vi "Drive Controller.vi"(8 "error in":errorcluster) -> ()   [LabVIEW 2018]
doc: "This VI executes continuously carrying out the current operation and responding to updates or new operation requests. It will often contain the timing or control code that is difficult to place directly in TeleOp. This VI generally opens all sensors and motors and isolates the rest of the robot code from knowing implementation details of how the operations are carried out."
uses:
  <vilib>/Rock Robotics/WPI/Framework/Completion Status.ctl
  Drive Setpoints.ctl
  Drive Operations.ctl
  Dawgma Programming Library/Controls/PurePursuit/RobotNeededPathData.ctl
  <vilib>/Rock Robotics/WPI/SafetyOutput/WPI_SafetyOutputConfigMenu.ctl
  <vilib>/Rock Robotics/SystemInterfaces/DIO/FPGA_DIOPWMChannel.ctl
  <vilib>/Rock Robotics/SystemInterfaces/DIO/FPGA_DIOChannel.ctl
  Logging/DataNames.ctl
  <vilib>/Rock Robotics/WPI/DriverStation/WPI_DriverStationRobotMode2.ctl
  <extravilib>/ChannelInstances/Lossy Stream-c(dbl,dbl,dbl,c(dbl,dbl))/Write With Abort.vi
  <extravilib>/ChannelInstances/Lossy Stream-c(dbl,dbl,dbl,c(dbl,dbl))/Read With Abort.vi
  <extravilib>/ChannelInstances/Lossy Stream-c(dbl,dbl,dbl,c(dbl,dbl))/Endpoint.vi
  <extravilib>/ChannelInstances/Lossy Stream-c(dbl,dbl,dbl,c(dbl,dbl))/EndpointRead.vi
  <vilib>/Rock Robotics/WPI/RobotDrive/WPI_RobotDriveOpen4MotorWithSPARK.vi
  <vilib>/Rock Robotics/WPI/Counter/WPI_CounterDigitalInputToDigitalSource.vi
  <vilib>/Rock Robotics/WPI/RobotDrive/WPI_RobotDriveOpen2MotorWithSPARK.vi
  <extravilib>/ChannelInstances/Lossy Stream-c(dbl,dbl,dbl,c(dbl,dbl))/Instantiate.vi
  Framework/Robot Global Data.vi
  <extravilib>/ChannelInstances/Lossy Stream-c(dbl,dbl,dbl,c(dbl,dbl))/)Channel.vi
  <resource>/ChannelSupport/_ChannelSupport/WaitIfNeeded.vi
  <vilib>/addons/control/pid/pid.llb/PID (DBL).vi
  Configuration/Constants.vi
  Drive Published Globals.vi
  <vilib>/Rock Robotics/Network Tables/NT Read Number.vi
  <vilib>/Rock Robotics/Network Tables/NT Write Number.vi
  <vilib>/addons/control/pid/NI_PID_pid.lvlib
  <extravilib>/ChannelInstances/Lossy Stream-c(dbl,dbl,dbl,c(dbl,dbl)).lvlib
panel:
  in  "Integral Range":dbl=15.0
  out "PID Tuining":cluster{dbl, dbl}(graph)={170.0, 167.02}
  in  "Points":cluster{"X":dbl, "Y":dbl}[](array[cluster])=[{"X"=0.0, "Y"=0.0}, {"X"=0.01, "Y"=0.0}, {"X"=0.011, "Y"=0.17}, {"X"=1.0, "Y"=1.0}]
  in  "PID gains":T1={"proportional gain (Kc)"=0.01, "integral time (Ti, min)"=0.007, "derivative time (Td, min)"=0.0015} {"derivative time (Td, min)" format="%#_9g"}
  in  "Gains":T2={"FFV"=0.0059, "FFA"=0.0019, "Vel PID"={"P"=0.01, "I"=0.0, "D"=0.0}}
  in  "Interactive Values":T3={"Operation"=enum."Turn to Angle", "Left Speed"=-0.27, "Right Speed"=0.27, "Duration"=2.0, "Speed"=0.0, "Start Angle"=0.0, "Target Angle"=180.0, "Distance (inch)"=0.0, "Start Point (inch)"=0.0, "RobotNeededPathData"={"Path"=[], "MaxVel"=0.0, "MaxAccel"=-1.0, "Backwards?"=FALSE, "PointSpacing"=0.0, "LookaheadDist"=0.0, "Speed/Curve"=1.8, "SlowDistanceAtEnd"=12.0, "SlowSpeed"=15.0, "MaxDeAccel"=0.0}, "Start Point 2"=0.0} {"RobotNeededPathData"."SlowSpeed" format="%#_13g"; "RobotNeededPathData"."SlowDistanceAtEnd" format="%#_13g"; "RobotNeededPathData"."Speed/Curve" format="%#_13g"}
  in  "Buttons":cluster{"Execute Cmd":bool, "Abort Cmd":bool}
  out "Command Timing":cluster{"Start Time (ms)":u32, "Iterations":i32}={"Start Time (ms)"=372507, "Iterations"=0}
  out "Status":T6
  out "Setpoints":T7(graph)
  out "Current\nCmd":string="Started at  14:51:47.884\nDefault: Reserve,  L 0.0, R 0.0, D 0.000000"
  # "Tip: The graph shows the motor setpoints. It may also be helpful to observe inputs and sensor values.\nYou may also want to display tuning or debugging controls."
  # "Interactive Command: You may fill in the settings for a command\nand schedule it with the Execute button. You can observe and abort\nany command while fine tuning the code for the controller."
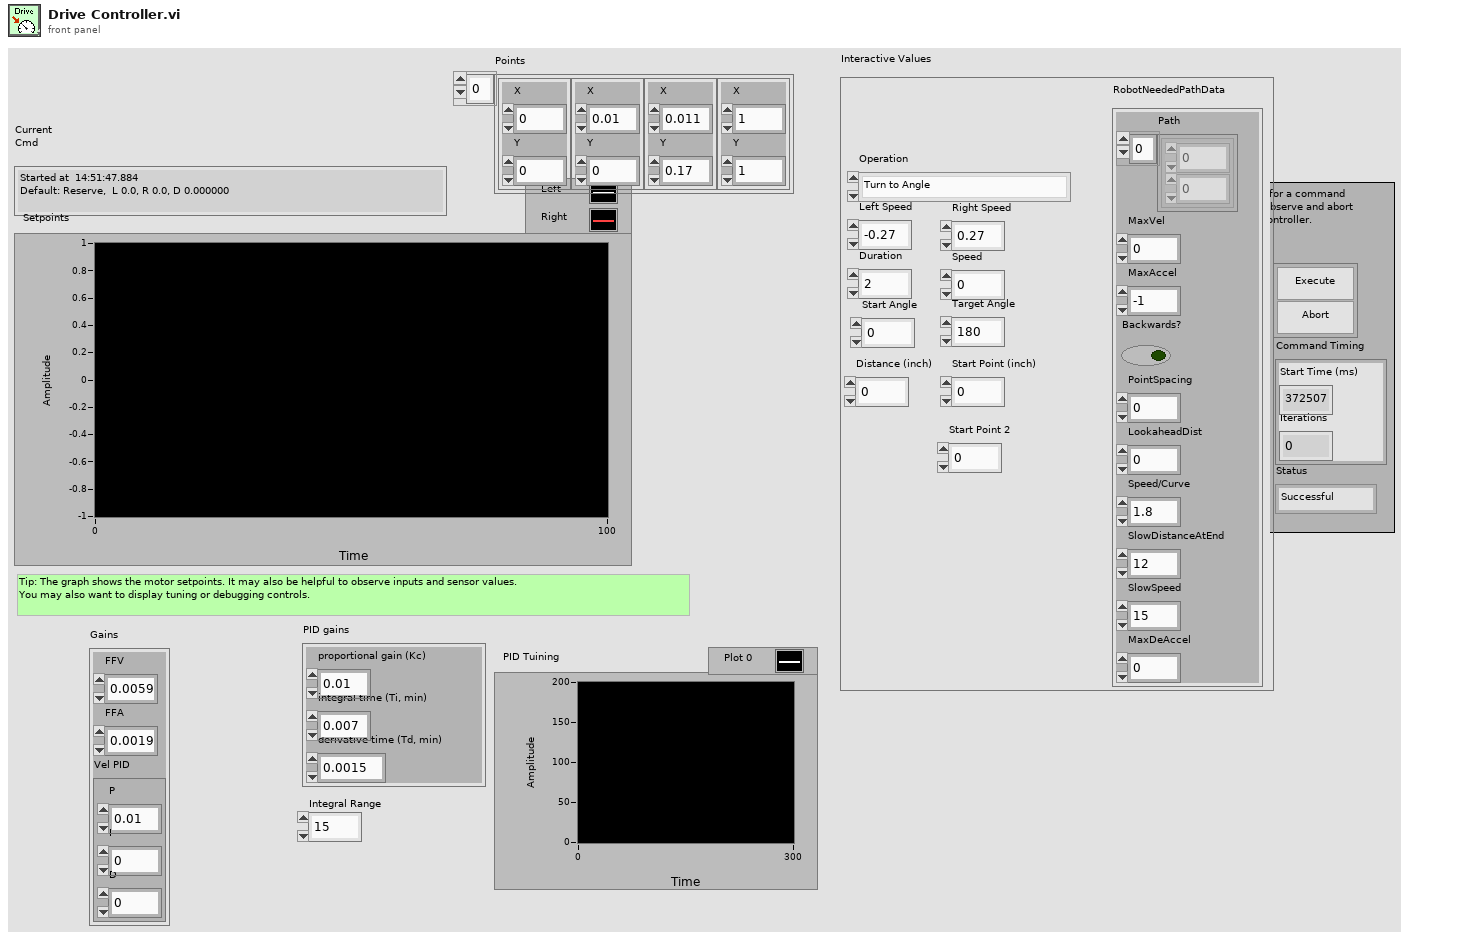
[diagram p1: front panel]
types:
  T1 = cluster{"proportional gain (Kc)":dbl, "integral time (Ti, min)":dbl, "derivative time (Td, min)":dbl}
  T2 = cluster{"FFV":dbl, "FFA":dbl, "Vel PID":cluster{"P":dbl, "I":dbl, "D":dbl}}
  T3 = typedef "Drive Setpoints.ctl" = cluster{"Operation":T4, "Left Speed":dbl, "Right Speed":dbl, "Duration":dbl, "Speed":dbl, "Start Angle":dbl, "Target Angle":dbl, "Distance (inch)":dbl, "Start Point (inch)":dbl, "RobotNeededPathData":T5, "Start Point 2":dbl}
  T4 = typedef "Drive Operations.ctl" = enum16{"Reserve", "Read Current", "Immediate", "Drive for Time", "Drive for Distance", "Turn to Angle", "Drive Path"}
  T5 = typedef "RobotNeededPathData.ctl" = cluster{"Path":cluster{dbl, dbl}[], "MaxVel":dbl, "MaxAccel":dbl, "Backwards?":bool, "PointSpacing":dbl, "LookaheadDist":dbl, "Speed/Curve":dbl, "SlowDistanceAtEnd":dbl, "SlowSpeed":dbl, "MaxDeAccel":dbl}
  T6 = typedef "Completion Status.ctl" = enum16{"Successful", "Aborted", "Incomplete"}
  T7 = cluster{"Left Setpoint":dbl, "Right Setpoint":dbl}
  T8 = typedef "DataNames.ctl" = enum16{"RobotMode", "FMSConnected", "DriveLeft", "DriveRight", "EncoderLeft", "EncoderRight", "Angle", "LocationX", "LocationY", "CPU", "DriveOperation", "Battery"}
  T9 = typedef "FPGA_DIOChannel.ctl" = enum8{"DIO 0", "DIO 1", "DIO 2", "DIO 3", "DIO 4", "DIO 5", "DIO 6", "DIO 7", "DIO 8", "DIO 9", "DIO MXP 0", "DIO MXP 1", "DIO MXP 2", "DIO MXP 3", "DIO MXP 4", "DIO MXP 5", "DIO MXP 6", "DIO MXP 7", "DIO MXP 8", "DIO MXP 9", "DIO MXP 10", "DIO MXP 11", "DIO MXP 12", "DIO MXP 13", "DIO MXP 14", "DIO MXP 15", "SPI Port CS1", "SPI Port CS2", "SPI Port CS3", "SPI Port MISO", "SPI Port MOSI", "Invalid"}
  T10 = typedef "FPGA_DIOPWMChannel.ctl" = enum8{"PWM 0", "PWM 1", "PWM 2", "PWM 3", "PWM 4", "PWM 5", "PWM 6", "PWM 7", "PWM 8", "PWM 9", "PWM MXP 0", "PWM MXP 1", "PWM MXP 2", "PWM MXP 3", "PWM MXP 4", "PWM MXP 5", "PWM MXP 6", "PWM MXP 7", "PWM MXP 8", "PWM MXP 9", "Invalid"}
  T11 = typedef "WPI_SafetyOutputConfigMenu.ctl" = enum16{"Enable", "Disable"}
  T12 = typedef "WPI_DigitalInputDevRef.ctl" = cluster{"DevStatus":errorcluster, "DIO Channel":T9}
  T13 = typedef "FPGA_CounterEncoderSourceConvertionLVSourceType.ctl" = cluster{"DevStatus":errorcluster, "AnalogTriggerMode?":bool, "DigitalMode":cluster{"DIO Channel":T14}, "AnalogTriggerMode":cluster{"AnalogTriggerIndex":T15, "OutputType":T16}}
  T14 = typedef "FPGA_DIODigitalSourceChannel.ctl" = enum8{"DIO 0", "DIO 1", "DIO 2", "DIO 3", "DIO 4", "DIO 5", "DIO 6", "DIO 7", "DIO 8", "DIO 9", "DIO MXP 0", "DIO MXP 1", "DIO MXP 2", "DIO MXP 3", "DIO MXP 4", "DIO MXP 5", "DIO MXP 6", "DIO MXP 7", "DIO MXP 8", "DIO MXP 9", "DIO MXP 10", "DIO MXP 11", "DIO MXP 12", "DIO MXP 13", "DIO MXP 14", "DIO MXP 15", "SPI Port CS1", "SPI Port CS2", "SPI Port CS3", "SPI Port MISO", "SPI Port MOSI", "Disabled"}
  T15 = typedef "FPGA_AnalogTriggerIndex.ctl" = enum8{"Trig 0", "Trig 1", "Trig 2", "Trig 3", "Trig 4", "Trig 5", "Trig 6", "Trig 7", "Invalid"}
  T16 = typedef "FPGA_AnalogTriggerOutType.ctl" = enum16{"InWindow", "TriggerState", "Rising", "Falling"}
  T17 = typedef "WPI_EncoderDevRef.ctl" = cluster{"DevStatus":errorcluster, "EncoderIndex":T18, "CounterIndex":T19, "DistancePerCount":dbl, "Decoding Type":T20}
  T18 = typedef "FPGA_EncoderIdx.ctl" = enum8{"Enc 0", "Enc 1", "Enc 2", "Enc 3", "Enc 4", "Enc 5", "Enc 6", "Enc 7", "Invalid"}
  T19 = typedef "FPGA_CounterCtrSystemIndex.ctl" = enum8{"Ctr 0", "Ctr 1", "Ctr 2", "Ctr 3", "Ctr 4", "Ctr 5", "Ctr 6", "Ctr 7", "Invalid"}
  T20 = typedef "WPI_EncoderType.ctl" = enum16{"1x", "2x", "4x"}
  T21 = typedef "WPI_RobotDriveDevRef.ctl" = cluster{"DevStatus":errorcluster, "Motors[]":T22[], "Square Inputs":bool, "Max Output":dbl}
  T22 = typedef "WPI_MotorControlDeviceRef.ctl" = cluster{"DeviceStatus":errorcluster, "Type":T23, "PWM":cluster{"PWM Channel":T10, "DeadBand":T24}, "CAN":cluster{"Device Number":u8, "SetOutput VI Ref":variant, "GetOutput VI Ref":variant, "Enable VI Ref":variant, "Disable VI Ref":variant, "Data":variant}, "Invert":bool, "DIO PWM":cluster{"PWM \"Enable\" Channel":T10, "DIOChannel":T9, "PWM Rate":dbl}}
  T23 = typedef "WPI_MotorControlType.ctl" = enum16{"PWM", "CAN", "DIO PWM"}
  T24 = typedef "WPI_PWMDeadband.ctl" = cluster{"Name":string, "maxPositivePwm":i32, "minPositivePwm":i32, "centerPwm":i32, "maxNegativePwm":i32, "minNegativePwm":i32, "angularRange":u16}
  T25 = typedef "Command Status Info.ctl" = cluster{"Name":string, "Status":T6, "notifier out":T26}
  T26 = typedef "Completion Notifier.ctl" = refnum<notifier>
  T27 = cluster{"SubSystem Data":T3, cluster{"Start Time (ms)":u32, "Iterations":i32}, cluster{"Command Info":T25, "Description":string, "Default Command":T3, "queue out":refnum<queue>, "Subsystem Name":string}}
  T28 = cluster{"LeftVel":dbl, "RightVel":dbl, "Yaw":dbl, "Pos":cluster{"X":dbl, "Y":dbl}}
  T29 = typedef "WPI_DriverStationRobotMode2.ctl" = enum16{"Autonomous Disabled", "Autonomous Enabled", "Teleop Disabled", "Teleop Enabled", "Disconnected", "Finish", "Test Disabled", "Test Enabled", "Emergency Stopped"}
  T30 = cluster{"Yaw":dbl, "Roll":dbl, "Pitch":dbl, "Heading":dbl, "Fused Heading":dbl}
  T31 = typedef "Lossy Stream-c(dbl,dbl,dbl,c(dbl,dbl)).lvlib/)Channel.ctl" = refnum<queue>
  T32 = cluster{"LeftDistance":dbl, "RightDistance":dbl, "LeftVelocity":dbl, "RightVelocity":dbl, "Angle":dbl, "Location":cluster{dbl, dbl}}
  T33 = cluster{"dx/dt":dbl, "dx/dt":dbl, "Yaw":dbl, cluster{dbl, dbl}}
  T34 = cluster{"SubSystem Data":T3, cluster{"Start Time (ms)":u32, "Iterations":i32}, "Default Command Arguments":cluster{"Command Info":T25, "Description":string, "Default Command":T3, "queue out":refnum<queue>, "Subsystem Name":string}}
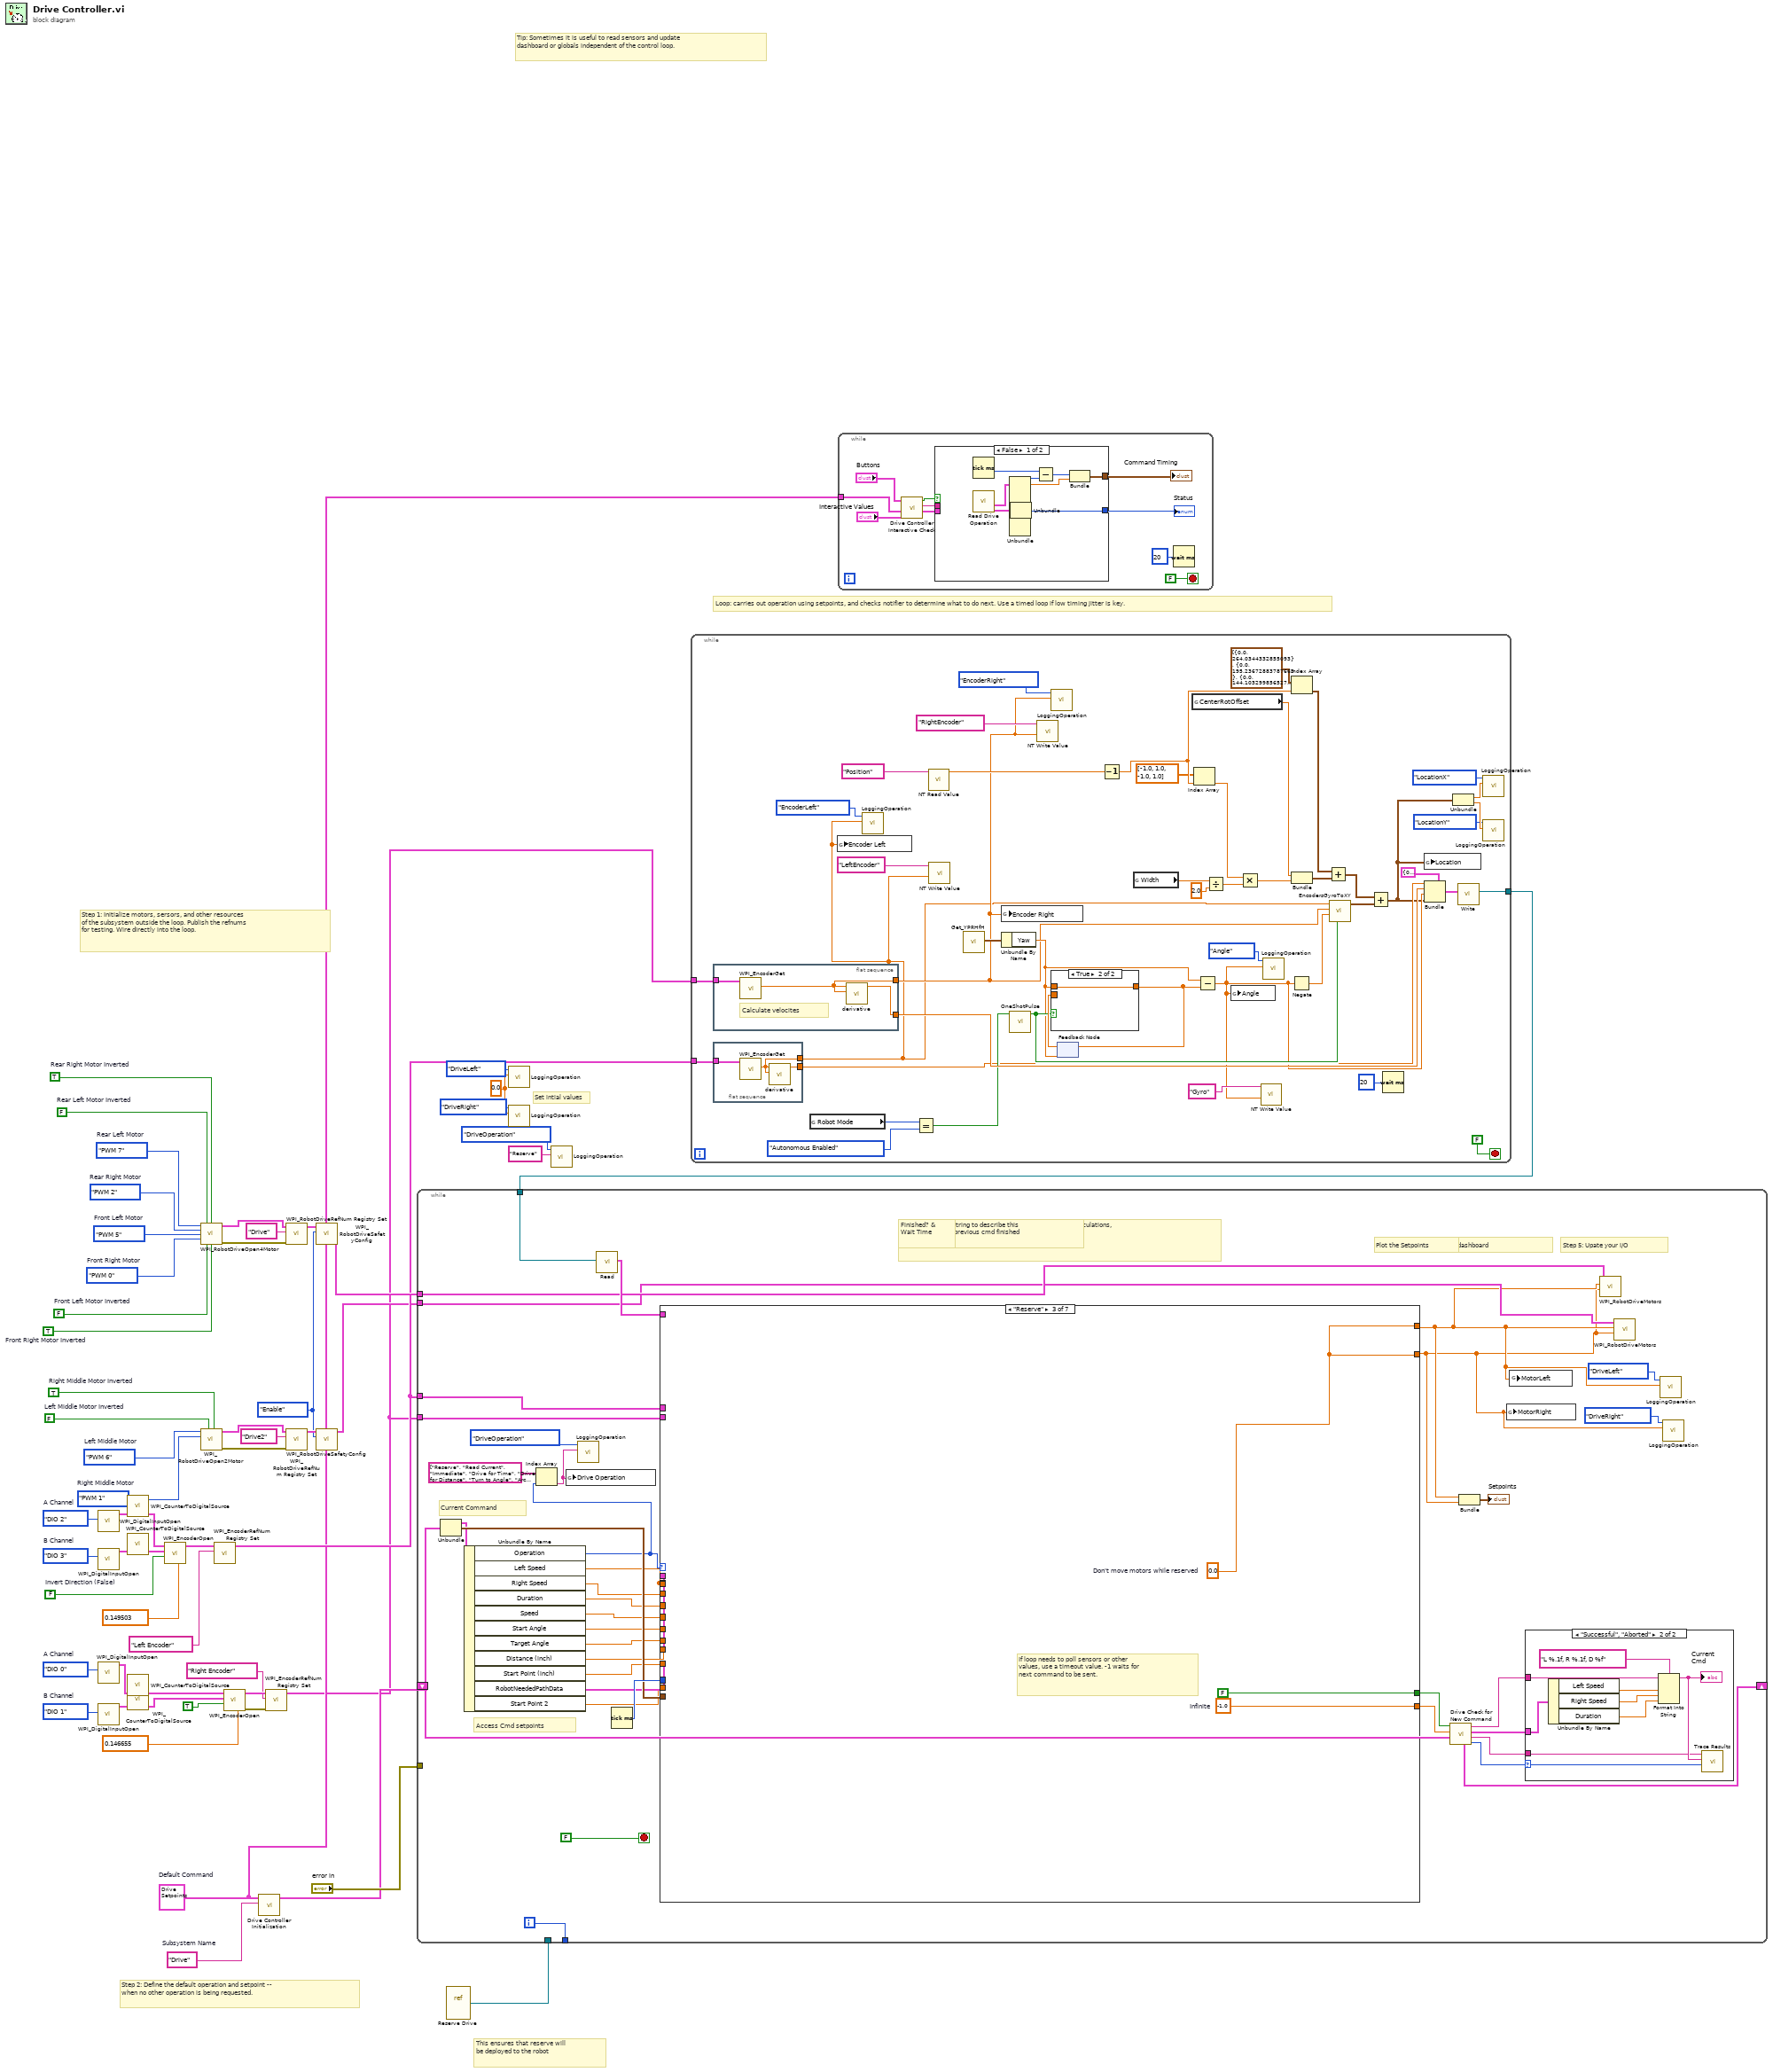
[diagram p0: block diagram]
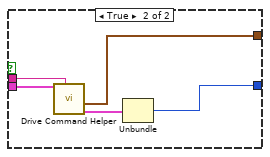
[diagram p3: hidden frame]
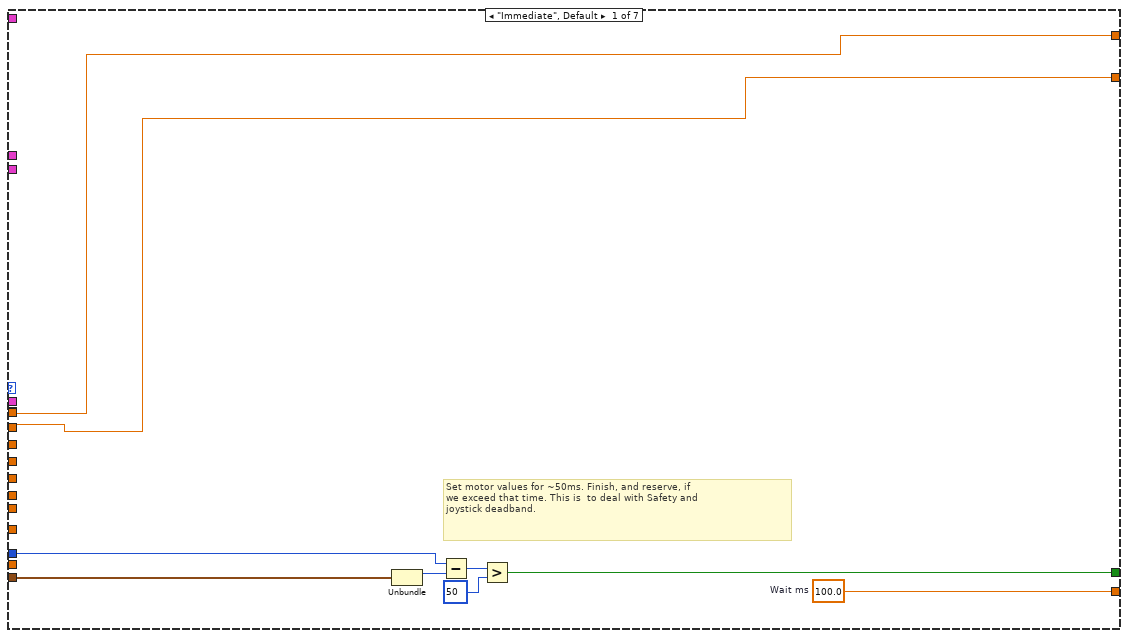
[diagram p4: hidden frame]
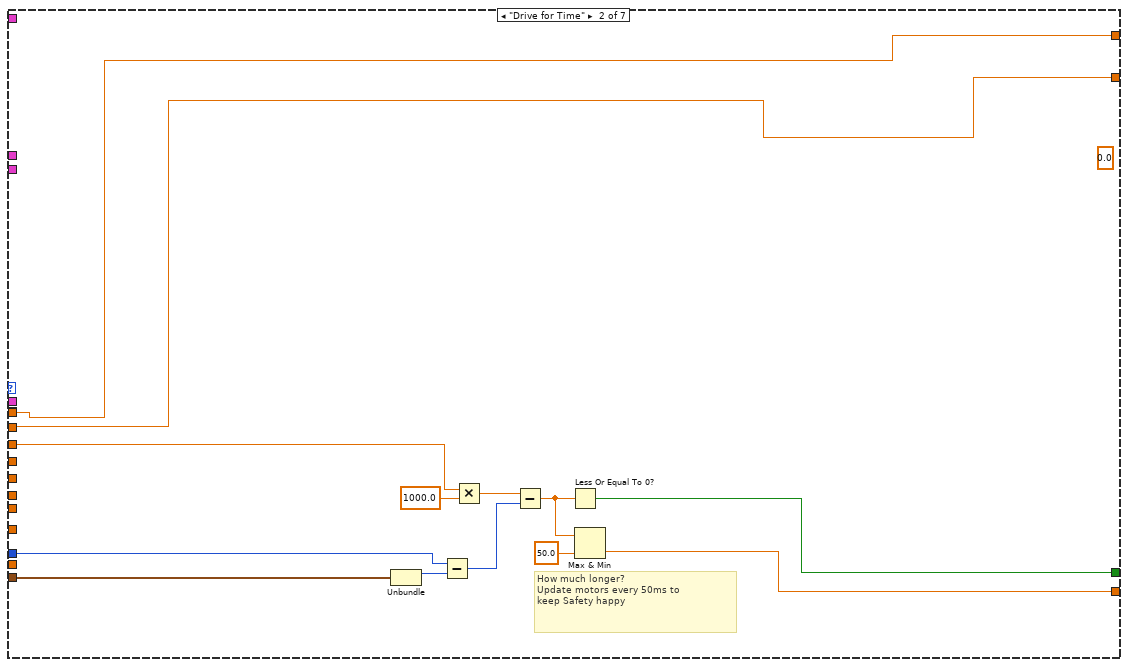
[diagram p5: hidden frame]
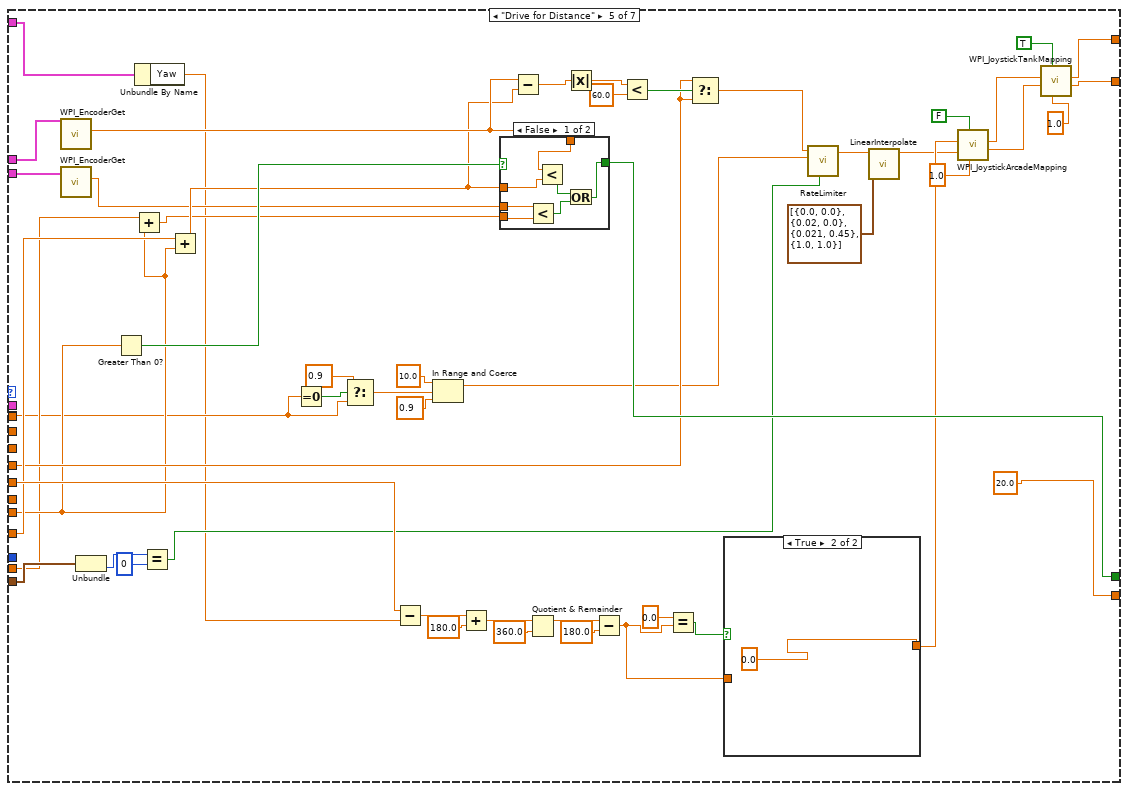
[diagram p7: hidden frame]
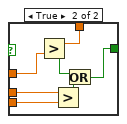
[diagram p8: hidden frame]
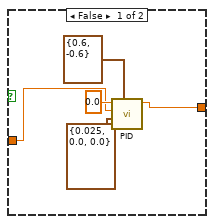
[diagram p9: hidden frame]
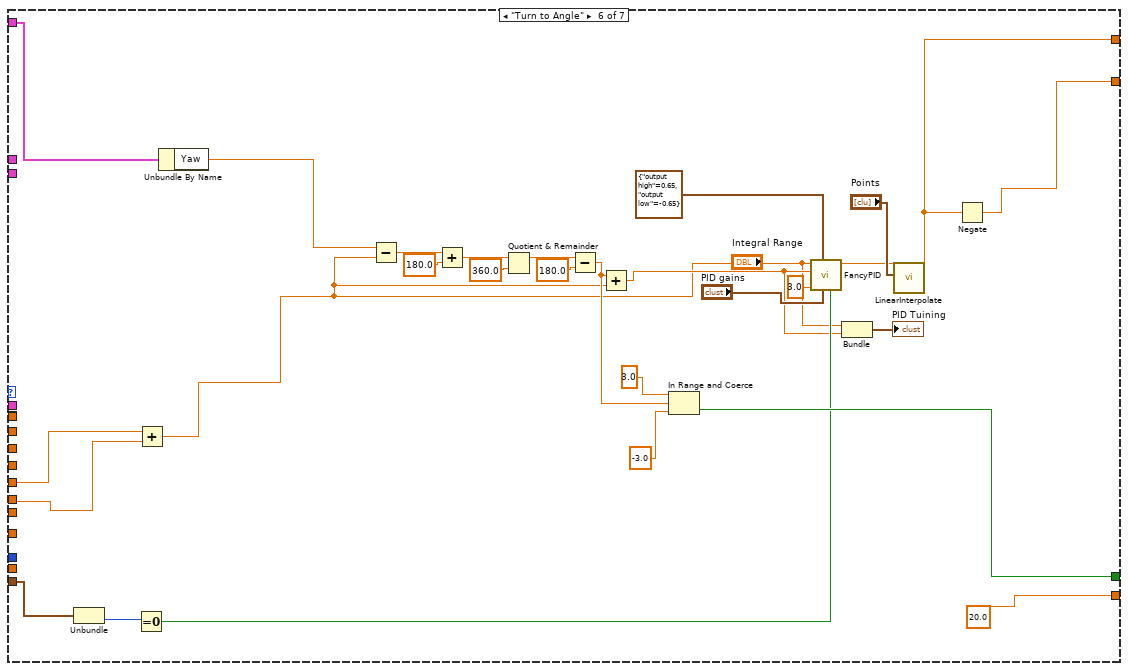
[diagram p10: hidden frame]
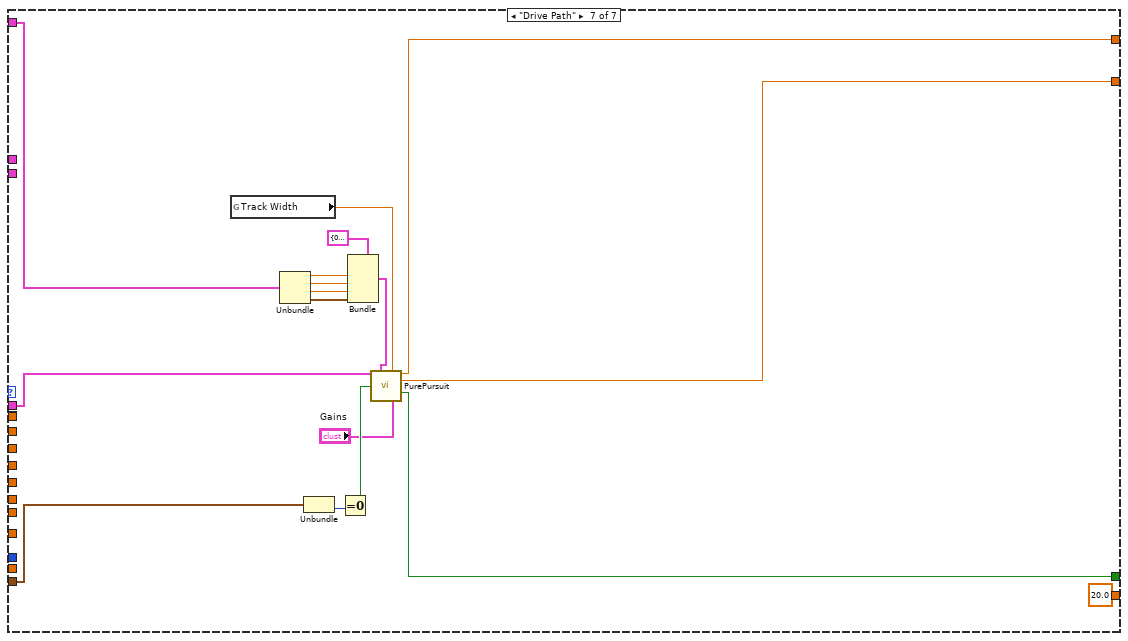
[diagram p11: hidden frame]
diagram:
  w2 = 0.0 ("y")
  w10 = FPGA_DIOChannel."DIO 1"  # B Channel
  w13 = FPGA_DIOChannel."DIO 0"  # A Channel
  w19 = T3 {"Operation"=enum."Reserve", "Left Speed"=0.0, "Right Speed"=0.0, "Duration"=0.0, "Speed"=0.0, "Start Angle"=0.0, "Target Angle"=0.0, "Distance (inch)"=0.0, "Start Point (inch)"=0.0, "RobotNeededPathData"={"Path"=[], "MaxVel"=0.0, "MaxAccel"=0.0, "Backwards?"=FALSE, "PointSpacing"=0.0, "LookaheadDist"=0.0, "Speed/Curve"=1.8, "SlowDistanceAtEnd"=12.0, "SlowSpeed"=15.0, "MaxDeAccel"=0.0}, "Start Point 2"=0.0}  # Default Command
  w26 = TRUE  # Right Middle Motor Inverted
  w27 = FALSE  # Left Middle Motor Inverted
  w30 = FPGA_DIOPWMChannel."PWM 1"  # Right Middle Motor
  w31 = FPGA_DIOPWMChannel."PWM 6"  # Left Middle Motor
  w40 = FALSE  # Invert Direction (False)
  w33 = FPGA_DIOChannel."DIO 3"  # B Channel
  w34 = FPGA_DIOChannel."DIO 2"  # A Channel
  w42 = TRUE  # Front Right Motor Inverted
  w43 = FALSE  # Front Left Motor Inverted
  w44 = TRUE  # Rear Right Motor Inverted
  w45 = FALSE  # Rear Left Motor Inverted
  w46 = FPGA_DIOPWMChannel."PWM 0"  # Front Right Motor
  w47 = FPGA_DIOPWMChannel."PWM 5"  # Front Left Motor
  w48 = FPGA_DIOPWMChannel."PWM 2"  # Rear Right Motor
  w49 = FPGA_DIOPWMChannel."PWM 7"  # Rear Left Motor
  w21 = WPI_SafetyOutputConfigMenu."Enable" ("mode")
  w57 = "Drive"  # Subsystem Name
  # "Set intial values"
  # "Step 1: Initialize motors, sersors, and other resources\nof the subsystem outside the loop. Publish the refnums\nfor testing. Wire directly into the loop."
  # "Step 2: Define the default operation and setpoint --\nwhen no other operation is being requested."
  # "This ensures that reserve will\nbe deployed to the robot"
  # "Tip: Sometimes it is useful to read sensors and update\ndashboard or globals independent of the control loop."
  # "Loop: carries out operation using setpoints, and checks notifier to determine what to do next. Use a timed loop if low timing jitter is key."
  n1 = call <vilib>:"WPI_DigitalInputOpen.vi"("DIO Channel"=w34) -> ("DigitalInputDevRef"=w37:T12)  [unwired: 1 in, 9 out]
  n2 = call <vilib>:"WPI_DigitalInputOpen.vi"("DIO Channel"=w33) -> ("DigitalInputDevRef"=w36:T12)  [unwired: 1 in, 9 out]
  n3 = call <vilib>:"WPI_DigitalInputOpen.vi"("DIO Channel"=w13) -> ("DigitalInputDevRef"=w14:T12)  [unwired: 1 in, 9 out]
  n4 = call <vilib>:"WPI_DigitalInputOpen.vi"("DIO Channel"=w10) -> ("DigitalInputDevRef"=w11:T12)  [unwired: 1 in, 9 out]
  n5 = call-poly <vilib>:"WPI_CounterToDigitalSource.vi"("DigitalInputDevRef"=w37) -> ("Digital Source"=w38:T13)  [unwired: 6 out]
  n6 = call-poly <vilib>:"WPI_CounterToDigitalSource.vi"("DigitalInputDevRef"=w36) -> ("Digital Source"=w35:T13)  [unwired: 6 out]
  n7 = call-poly <vilib>:"WPI_CounterToDigitalSource.vi"("DigitalInputDevRef"=w14) -> ("Digital Source"=w15:T13)  [unwired: 6 out]
  n8 = call-poly <vilib>:"WPI_CounterToDigitalSource.vi"("DigitalInputDevRef"=w11) -> ("Digital Source"=w12:T13)  [unwired: 6 out]
  n9 = call <vilib>:"WPI_EncoderOpen.vi"("DistancePerCount"=0.149503, "Invert Direction (False)"=w40, "BSource"=w35, "ASource"=w38) -> ("EncoderDevRef"=w39:T17)  [unwired: 4 in, 3 out]
  n10 = call-poly <vilib>:"WPI_RobotDriveOpen4Motor.vi"("Rear Left Motor"=w49, "Rear Left Motor Inverted"=w45, "Rear Right Motor Inverted"=w44, "Rear Right Motor"=w48, "Front Left Motor"=w47, "Front Right Motor"=w46, "Front Left Motor Inverted"=w43, "Front Right Motor Inverted"=w42) -> ("RobotDriveDevRef"=w56:T21, "error out"=w54:errorcluster)  [unwired: 6 in]
  n11 = call-poly <vilib>:"WPI_RobotDriveOpen2Motor.vi"("Right Motor Inverted"=w26, "Left Motor Inverted"=w27, "Right Motor"=w30, "Left Motor"=w31) -> ("error out"=w25:errorcluster, "RobotDriveDevRef"=w29:T21)  [unwired: 6 in]
  n12 = call <vilib>:"WPI_EncoderRefNum Registry Set.vi"("refnum name"="Left Encoder", "EncoderDevRef"=w39) -> ("EncoderDevRef"=w32:T17)  [unwired: 8 in, 1 out]
  n13 = call <vilib>:"WPI_EncoderOpen.vi"("DistancePerCount"=0.146655, "Invert Direction (False)"=TRUE, "BSource"=w12, "ASource"=w15) -> ("error out"=w17:errorcluster, "EncoderDevRef"=w16:T17)  [unwired: 4 in, 2 out]
  n14 = call "Drive Controller Initialization.vi"("Subsystem Name"=w57, "Default Command"=w19) -> ("Current Command"=w51:T27)  [unwired: 9 in]
  n15 = call <vilib>:"WPI_EncoderRefNum Registry Set.vi"("error in (no error)"=w17, "refnum name"="Right Encoder", "EncoderDevRef"=w16) -> ("EncoderDevRef"=w18:T17)  [unwired: 7 in, 1 out]
  n16 = call <vilib>:"WPI_RobotDriveRefNum Registry Set.vi"("error in (no error)"=w54, "refnum name"="Drive", "RobotDriveDevRef"=w56) -> ("RobotDriveDevRef"=w24:T21)  [unwired: 1 in, 7 out]
  n17 = call <vilib>:"WPI_RobotDriveRefNum Registry Set.vi"("error in (no error)"=w25, "refnum name"="Drive2", "RobotDriveDevRef"=w29) -> ("RobotDriveDevRef"=w23:T21)  [unwired: 7 in, 1 out]
  n18 = call <vilib>:"WPI_RobotDriveSafetyConfig.vi"("mode"=w21, "RobotDriveDevRef"=w24) -> ("RobotDriveDevRef"=w53:T21)  [unwired: 8 in, 1 out]
  n19 = call <vilib>:"WPI_RobotDriveSafetyConfig.vi"("mode"=w21, "RobotDriveDevRef"=w23) -> ("RobotDriveDevRef"=w22:T21)  [unwired: 8 in, 1 out]
  n20 = vi-ref "Reserve Drive.vi"() -> (w50:refnum<vi>)
  n21 = call "LoggingOperation.vi"("Data"=w2, "Name"=DataNames."DriveLeft") -> ()  [unwired: 9 in, 1 out]
  n22 = call "LoggingOperation.vi"("Data"=w2, "Name"=DataNames."DriveRight") -> ()  [unwired: 9 in, 1 out]
  n23 = call "LoggingOperation.vi"("Data"="Reserve", "Name"=DataNames."DriveOperation") -> ()  [unwired: 9 in, 1 out]
  n24 = while {
    tunnel: w18 -> [w80]
    tunnel: w32 -> [w79]
    tunnel: [w59] -> w1
    stop <- FALSE stop-if-true
    n25 = flat-sequence {
      tunnel: [w111] -> w101
      tunnel: [w110] -> w71
      tunnel: w80 -> [w112]
      frame #0 {
        # "Calculate velocites"
        n26 = call <vilib>:"WPI_EncoderGet.vi"("EncoderDevRef"=w112) -> ("Distance"=w110:dbl)  [unwired: 5 in, 5 out]
        n27 = call "derivative.vi"("Starting value"=w110, "x"=w110) -> ("dx/dt"=w111:dbl)  [unwired: 9 in]
      }
    }
    n28 = flat-sequence {
      tunnel: [w107] -> w81
      tunnel: [w106] -> w70
      tunnel: w79 -> [w105]
      frame #0 {
        n29 = call <vilib>:"WPI_EncoderGet.vi"("EncoderDevRef"=w105) -> ("Distance"=w106:dbl)  [unwired: 5 in, 5 out]
        n30 = call "derivative.vi"("Starting value"=w106, "x"=w106) -> ("dx/dt"=w107:dbl)  [unwired: 9 in]
      }
    }
    n31 = global read "Robot Global Data.vi" "Robot Mode"() -> (w94:T29)
    n32 = global write "Drive Published Globals.vi" "Encoder Left"(w70) -> ()
    n33 = call "LoggingOperation.vi"("Data"=w70, "Name"=DataNames."EncoderLeft") -> ()  [unwired: 9 in, 1 out]
    n34 = Equal?(x=w94, y=WPI_DriverStationRobotMode2."Autonomous Enabled") -> (x = y?=w95:bool)
    n35 = call-poly <vilib>:"NT Read Value.vi"("Name"="Position") -> ("Numeric"=w77:dbl)  [unwired: 9 in, 1 out]
    n36 = call-poly <vilib>:"NT Write Value.vi"("Numeric"=w70, "Name"="LeftEncoder") -> ()  [unwired: 9 in, 1 out]
    n37 = call <vilib>:"Get_YPRHfH.vi"() -> ("YRPHfH"=w104:T30)  [unwired: 11 in]
    n38 = global write "Drive Published Globals.vi" "Encoder Right"(w71) -> ()
    n39 = Unbundle By Name(w104) -> ("Yaw"=w73:dbl)
    n40 = call "OneShotPulse.vi"("Input"=w95) -> ("Output"=w96:bool)  [unwired: 10 in]
    n41 = call-poly <vilib>:"NT Write Value.vi"("Numeric"=w71, "Name"="RightEncoder") -> ()  [unwired: 9 in, 1 out]
    n42 = call "LoggingOperation.vi"("Data"=w71, "Name"=DataNames."EncoderRight") -> ()  [unwired: 9 in, 1 out]
    n43 = feedback #1(w73) -> (w97:dbl)
    n44 = case shown="True" w96 {
      tunnel: w73 -> [_ w109]
      tunnel: [w108 w109] -> w98
      tunnel: w97 -> [w108 _]
      frame False {
      }
      frame True {
      }
    }
    n45 = feedback-in #1(w98) -> ()
    n46 = Decrement(x=w77) -> (x-1=w89:dbl)
    n47 = global read "Constants.vi" "Width"() -> (w84:dbl)
    n48 = global read "Constants.vi" "CenterRotOffset"() -> (w82:dbl)
    n49 = Index Array(array=dbl[] [-1.0, 1.0, -1.0, 1.0], index=w89) -> (element=w90:dbl)
    n50 = Subtract(x=w73, y=w98) -> (x-y=w62:dbl)
    n51 = Divide(x=w84, y=2.0) -> (x/y=w85:dbl)
    n52 = global write "Drive Published Globals.vi" "Angle"(w62) -> ()
    n53 = Multiply(x=w90, y=w85) -> (x*y=w91:dbl)
    n54 = call-poly <vilib>:"NT Write Value.vi"("Numeric"=w62, "Name"="Gyro") -> ()  [unwired: 9 in, 1 out]
    n55 = call "LoggingOperation.vi"("Data"=w62, "Name"=DataNames."Angle") -> ()  [unwired: 9 in, 1 out]
    n56 = Negate(x=w62) -> (-x=w99:dbl)
    n57 = Index Array(array=cluster{dbl, dbl}[] [{0.0, 264.0344332855093}, {0.0, 195.23672883787663}, {0.0, 144.10329985652797}, {0.0, -0.0}] ("x*y"), index=w89) -> (element=w88:cluster{dbl, dbl})
    n58 = Bundle("CenterRotOffset"=w82, w91) -> (w92:cluster{"CenterRotOffset":dbl, dbl})  [unwired: 1 in]
    n59 = Add(x=w88, y=w92) -> (x+y=w69:cluster{dbl, dbl})
    n60 = call "EncodersGyroToXY.vi"("Reset"=w96, "Angle (degrees)"=w99, "Right Distance"=w71, "Left Distance"=w70) -> ("Location"=w100:cluster{dbl, dbl})  [unwired: 7 in]
    n61 = Add(x=w69, y=w100) -> (x+y=w58:cluster{dbl, dbl})
    n62 = Wait (ms)(milliseconds to wait=u32 20) -> ()  [unwired: 1 out]
    n63 = global write "Drive Published Globals.vi" "Location"(w58) -> ()
    n64 = Bundle(cluster=T28 {"LeftVel"=0.0, "RightVel"=0.0, "Yaw"=0.0, "Pos"={"X"=0.0, "Y"=0.0}} ("Robot"), "LeftVel"=w81, "RightVel"=w101, "Yaw"=w62, "Pos"=w58) -> (w60:T28)
    n65 = Unbundle(w58) -> (w68:dbl, w67:dbl)
    n66 = call <extravilib>:"Write.vi"("element"=w60) -> ("channel"=w59:T31)  [unwired: 8 in, 2 out]
    n67 = call "LoggingOperation.vi"("Data"=w68, "Name"=DataNames."LocationX") -> ()  [unwired: 9 in, 1 out]
    n68 = call "LoggingOperation.vi"("Data"=w67, "Name"=DataNames."LocationY") -> ()  [unwired: 9 in, 1 out]
  }
  n69 = while {
    shift-right: [w146] -> _
    shift-left: w51 -> [w119]
    tunnel: [w149] -> _
    tunnel: w53 -> [w126]
    tunnel: "error in" -> [_]
    tunnel: w50 -> [_]
    tunnel: w32 -> [w124]
    tunnel: w22 -> [w125]
    tunnel: w1 -> [w128]
    tunnel: w18 -> [w123]
    i -> [w149]
    stop <- FALSE stop-if-true
    # "Plot the Setpoints"
    # "Step 5: Upate your I/O"
    # "Step 4: Format a string to describe this\ncmd and how the previous cmd finished"
    # "Current Command"
    # "Update motors and update dashboard"
    # "Access Cmd setpoints"
    # "Finished? &\nWait Time"
    # "Step 3: For a given operation, read from sensors, perform calculations,\nupdate actuators and status.\nOperations can be merged to a single case."
    n70 = Unbundle(w119) -> ("SubSystem Data"=w129:T3, w140:cluster{"Start Time (ms)":u32, "Iterations":i32})  [unwired: 1 out]
    n71 = Unbundle By Name(w129) -> ("Operation"=w121:T4, "Left Speed"=w138:dbl, "Right Speed"=w137:dbl, "Duration"=w136:dbl, "Speed"=w135:dbl, "Start Angle"=w134:dbl, "Target Angle"=w133:dbl, "Distance (inch)"=w132:dbl, "Start Point (inch)"=w131:dbl, "RobotNeededPathData"=w130:T5, "Start Point 2"=w122:dbl)
    n72 = Index Array(array=string[] ["Reserve", "Read Current", "Immediate", "Drive for Time", "Drive for Distance", "Turn to Angle", "Arc Turn", "Drive Path", "Drive To Cube"] ("Strings []"), index=w121) -> (element=w114:string)
    n73 = global write "Robot Global Data.vi" "Drive Operation"(w114) -> ()
    n74 = call "LoggingOperation.vi"("Data"=w114, "Name"=DataNames."DriveOperation") -> ()  [unwired: 9 in, 1 out]
    n75 = call <extravilib>:"Read.vi"("channel"=w128) -> ("element"=w127:T33)  [unwired: 5 in, 5 out]
    n76 = Tick Count (ms)() -> (millisecond timer value=w148:u32)
    n77 = case shown="\"Reserve\"" w121 {
      tunnel: [w159 w163 w175 _ 20.0 ("Infinite") 20.0 ("Infinite") 20.0 ("Infinite")] -> w145
      tunnel: [w154 w167 FALSE ("ignore previous (F)") _ w219 w272 w291] -> w144
      tunnel: w140 -> [w153 w169 _ _ w201 w263 w281]
      tunnel: w148 -> [w155 w166 _ _ _ _ _]
      tunnel: [w152 w161 w173 _ w206 w261 w293] -> w118
      tunnel: [w151 w160 w173 _ w207 w260 w292] -> w117
      tunnel: w135 -> [_ _ _ _ w190 _ _]
      tunnel: w132 -> [_ _ _ _ w188 _ _]
      tunnel: w136 -> [_ w162 _ _ _ _ _]
      tunnel: w138 -> [w152 _ _ _ w182 _ _]
      tunnel: w137 -> [w151 w160 _ _ _ _ _]
      tunnel: w124 -> [_ _ _ _ w217 _ _]
      tunnel: w134 -> [_ _ _ _ w213 w275 _]
      tunnel: w133 -> [_ _ _ _ _ w274 _]
      tunnel: w131 -> [_ _ _ _ w212 _ _]
      tunnel: w138 -> [_ w161 _ _ _ _ _]
      tunnel: w130 -> [_ _ _ _ _ _ w294]
      tunnel: w127 -> [_ _ _ _ w177 w250 w285]
      tunnel: w123 -> [_ _ _ _ w189 _ _]
      tunnel: w122 -> [_ _ _ _ w187 _ _]
      frame "Immediate", Default {
        w159 = 100.0  # Wait ms
        # "Set motor values for ~50ms. Finish, and reserve, if\nwe exceed that time. This is  to deal with Safety and\njoystick deadband."
        n78 = Unbundle(w153) -> ("Start Time (ms)"=w156:u32)  [unwired: 1 out]
        n79 = Subtract(x=w155, y=w156) -> (x-y=w157:u32)
        n80 = Greater?(x=w157, y=u8 50 ("Left Motor")) -> (0:w154:bool)
      }
      frame "Drive for Time" {
        (unwired) 0.0 ("output")
        # "How much longer?\nUpdate motors every 50ms to\nkeep Safety happy"
        n81 = Unbundle(w169) -> ("Start Time (ms)"=w168:u32)  [unwired: 1 out]
        n82 = Subtract(x=w166, y=w168) -> (x-y=w172:u32)
        n83 = Multiply(x=w162, y=1000.0) -> (x*y=w171:dbl)
        n84 = Subtract(x=w171, y=w172) -> (x-y=w165:dbl)
        n85 = Less Or Equal To 0?(x=w165) -> (x <= 0?=w167:bool)
        n86 = Max & Min(x=w165, y=50.0) -> (min(x,y)=w163:dbl)  [unwired: 1 out]
      }
      frame "Reserve" {
        w173 = 0.0  # Don't move motors while reserved
        w175 = -1.0  # Infinite
        # "If loop needs to poll sensors or other\nvalues, use a timeout value. -1 waits for\nnext command to be sent."
      }
      frame "Read Current" {
      }
      frame "Drive for Distance" {
        n87 = call <vilib>:"WPI_EncoderGet.vi"("EncoderDevRef"=w217) -> ("Distance"=w197:dbl)  [unwired: 5 in, 5 out]
        n88 = call <vilib>:"WPI_EncoderGet.vi"("EncoderDevRef"=w189) -> ("Distance"=w185:dbl)  [unwired: 5 in, 5 out]
        n89 = Unbundle(w201) -> ("Iterations"=w200:i32)  [unwired: 1 out]
        n90 = Greater Than 0?(x=w188) -> (x > 0?=w211:bool)
        n91 = Add(x=w187, y=w188) -> (x+y=w186:dbl)
        n92 = Unbundle By Name(w177) -> ("Yaw"=w176:dbl)
        n93 = Equal?(x=w200, y=0) -> (x = y?=w198:bool)
        n94 = Add(x=w212, y=w188) -> (x+y=w196:dbl)
        n95 = Equal To 0?(x=w182) -> (x = 0?=w184:bool)
        n96 = Select(t=0.9, s=w184, f=w182) -> (s? t:f=w181:dbl)
        n97 = Subtract(x=w213, y=w176) -> (x-y=w221:dbl)
        n98 = In Range and Coerce(upper limit=10.0, x=w181, lower limit=0.9) -> (coerced(x)=w178:dbl)  [unwired: 1 out]
        n99 = Add(x=w221, y=180.0) -> (x+y=w225:dbl)
        n100 = case shown="False" w211 {
          tunnel: w197 -> [w234 w242]
          tunnel: w196 -> [w235 w241]
          tunnel: [w232 w236] -> w219
          tunnel: w186 -> [w230 w240]
          tunnel: w185 -> [w231 w239]
          frame False {
            n101 = Less?(x=w231, y=w230) -> (x < y?=w229:bool)
            n102 = Less?(x=w234, y=w235) -> (x < y?=w233:bool)
            n103 = Or(x=w233, y=w229) -> (x .or. y?=w232:bool)
          }
          frame True {
            n104 = Greater?(x=w242, y=w241) -> (0:w238:bool)
            n105 = Greater?(x=w239, y=w240) -> (0:w237:bool)
            n106 = Or(x=w238, y=w237) -> (x .or. y?=w236:bool)
          }
        }
        n107 = Subtract(x=w197, y=w196) -> (x-y=w195:dbl)
        n108 = Quotient & Remainder(x=w225, y=360.0) -> (x-y*floor(x/y)=w223:dbl)  [unwired: 1 out]
        n109 = Absolute Value(x=w195) -> (abs(x)=w194:dbl)
        n110 = Subtract(x=w223, y=180.0) -> (x-y=w220:dbl)
        n111 = Less?(x=w194, y=60.0) -> (x < y?=w192:bool)
        n112 = Equal?(x=0.0, y=w220) -> (x = y?=w228:bool)
        n113 = Select(t=w190, s=w192, f=w190) -> (s? t:f=w191:dbl)
        n114 = case shown="True" w228 {
          tunnel: [w243 0.0] -> w214
          tunnel: w220 -> [w244 _]
          frame False {
            n115 = call-poly <vilib>:"PID.vi"("output range"=cluster{"output high":dbl, "output low":dbl} {"output high"=0.6, "output low"=-0.6}, "PID gains"=T1 {"proportional gain (Kc)"=0.025, "integral time (Ti, min)"=0.0, "derivative time (Td, min)"=0.0}, "process variable"=w244, "setpoint"=0.0) -> ("output"=w243:dbl)  [unwired: 6 in, 1 out]
          }
          frame True {
          }
        }
        n116 = call "RateLimiter.vi"("Reset"=w198, "Max dx/dt"=w178, "Input"=w191) -> ("Output"=w209:dbl)  [unwired: 8 in]
        n117 = call "LinearInterpolate.vi"("Points"=cluster{"X":dbl, "Y":dbl}[] [{"X"=0.0, "Y"=0.0}, {"X"=0.02, "Y"=0.0}, {"X"=0.021, "Y"=0.45}, {"X"=1.0, "Y"=1.0}], "Value"=w209) -> ("Output"=w210:dbl)  [unwired: 9 in]
        n118 = call <vilib>:"WPI_JoystickArcadeMapping.vi"("Max Output"=1.0, "Square Inputs"=FALSE, "Y axis value"=w210, "X axis value"=w214) -> ("Right Motor Value"=w205:dbl, "Left Motor Value"=w204:dbl)  [unwired: 6 in]
        n119 = call <vilib>:"WPI_JoystickTankMapping.vi"("Max Output"=1.0, "Square Inputs"=TRUE, "Right axis value"=w205, "Left axis value"=w204) -> ("Right Motor Value"=w207:dbl, "Left Motor Value"=w206:dbl)  [unwired: 6 in]
      }
      frame "Turn to Angle" {
        n120 = Unbundle(w263) -> ("Iterations"=w262:i32)  [unwired: 1 out]
        n121 = Equal To 0?(x=w262) -> (x = 0?=w256:bool)
        n122 = Add(x=w275, y=w274) -> (x+y=w253:dbl)
        n123 = Unbundle By Name(w250) -> ("Yaw"=w249:dbl)
        n124 = Subtract(x=w249, y=w253) -> (x-y=w266:dbl)
        n125 = Add(x=w266, y=180.0) -> (x+y=w269:dbl)
        n126 = Quotient & Remainder(x=w269, y=360.0) -> (x-y*floor(x/y)=w267:dbl)  [unwired: 1 out]
        n127 = Subtract(x=w267, y=180.0) -> (x-y=w265:dbl)
        n128 = Add(x=w265, y=w253) -> (x+y=w254:dbl)
        n129 = In Range and Coerce(upper limit=3.0, x=w265, lower limit=-3.0) -> (In Range?=w272:bool)  [unwired: 1 out]
        n130 = call "FancyPID.vi"("Reset"=w256, "Gains"="PID gains", "Range"=cluster{"output high":dbl, "output low":dbl} {"output high"=0.65, "output low"=-0.65} ("output range"), "Disable Range"=3.0, "Integral Range"="Integral Range", "Process variable"=w254, "Setpoint"=w253) -> ("output"=w257:dbl)  [unwired: 4 in]
        n131 = Bundle(w253, w254) -> (→"PID Tuining":cluster{dbl, dbl})  [unwired: 1 in]
        n132 = call "LinearInterpolate.vi"("Points"="Points", "Value"=w257) -> ("Output"=w261:dbl)  [unwired: 9 in]
        n133 = Negate(x=w261) -> (-x=w260:dbl)
      }
      frame "Drive Path" {
        n134 = global read "Constants.vi" "Track Width"() -> (w280:dbl)
        n135 = Unbundle(w285) -> ("dx/dt"=w289:dbl, "dx/dt"=w288:dbl, "Yaw"=w287:dbl, w286:cluster{dbl, dbl})
        n136 = Unbundle(w281) -> ("Iterations"=w282:i32)  [unwired: 1 out]
        n137 = Equal To 0?(x=w282) -> (x = 0?=w283:bool)
        n138 = Bundle(cluster=T32 {"LeftDistance"=0.0, "RightDistance"=0.0, "LeftVelocity"=0.0, "RightVelocity"=0.0, "Angle"=0.0, "Location"={0.0, 0.0}} ("SensorData"), "LeftVelocity"=w289, "RightVelocity"=w288, "Angle"=w287, "Location"=w286) -> (w290:T32)  [unwired: 2 in]
        n139 = call "PurePursuit.vi"("RobotNeededPathData"=w294, "SensorData"=w290, "Trackwidth"=w280, "Reset"=w283, "Gains"="Gains") -> ("LeftValue"=w293:dbl, "RightValue"=w292:dbl, "Done"=w291:bool)  [unwired: 6 in, 2 out]
      }
    }
    n140 = call "Drive Check for New Command.vi"("input cluster"=w119, "Wait time (ms)"=w145, "Finished?"=w144) -> ("Completion"=w147:T6, "Subsystem Name"=w141:string, "Current Command"=w142:T3, "Initial Trace String"=w143:string, "Next Command"=w146:T34)  [unwired: 4 in]
    n141 = Bundle("LeftValue"=w118, "RightValue"=w117) -> (→"Setpoints":cluster{"LeftValue":dbl, "RightValue":dbl})  [unwired: 1 in]
    n142 = global write "Drive Published Globals.vi" "MotorRight"(w117) -> ()
    n143 = global write "Drive Published Globals.vi" "MotorLeft"(w118) -> ()
    n144 = case shown="\"Successful\", \"Aborted\"" w147 {
      selector: w147 -> [_ w303]
      tunnel: w143 -> [_ w298]
      tunnel: w142 -> [_ w299]
      tunnel: w141 -> [_ w295]
      frame "Incomplete", Default {
        # "Continuing current command"
      }
      frame "Successful", "Aborted" {
        # "Report and setup for next command"
        n145 = Unbundle By Name(w299) -> ("Left Speed"=w301:dbl, "Right Speed"=w302:dbl, "Duration"=w296:dbl)
        n146 = Format Into String(format string="L %.1f, R %.1f, D %f", initial string=w298, w301, w302, w296) -> (resulting string=w297:string)  [unwired: 1 in, 1 out]
        "Current\nCmd" <- w297
        n147 = call <vilib>:"Trace Results.vi"("Status of previous command"=w303, "Description"=w297, "Subsystem"=w295) -> ()  [unwired: 9 in]
      }
    }
    n148 = call <vilib>:"WPI_RobotDriveMotors.vi"("RightSpeed"=w117, "LeftSpeed"=w118, "RobotDriveDevRef"=w126) -> ()  [unwired: 1 in, 8 out]
    n149 = call <vilib>:"WPI_RobotDriveMotors.vi"("RightSpeed"=w117, "LeftSpeed"=w118, "RobotDriveDevRef"=w125) -> ()  [unwired: 1 in, 8 out]
    n150 = call "LoggingOperation.vi"("Data"=w118, "Name"=DataNames."DriveLeft") -> ()  [unwired: 9 in, 1 out]
    n151 = call "LoggingOperation.vi"("Data"=w117, "Name"=DataNames."DriveRight") -> ()  [unwired: 9 in, 1 out]
  }
  n152 = while {
    tunnel: w19 -> [w305]
    stop <- FALSE stop-if-true
    n153 = call "Drive Controller Interactive Check.vi"("Interactive Command In"="Interactive Values", "Default Command"=w305, "Buttons"="Buttons") -> ("Interactive Command Out"=w307:T3, "Trace String"=w308:string, "Schedule"=w309:bool)  [unwired: 6 in]
    n154 = case shown="False" w309 {
      tunnel: [w318 w326] -> w310
      tunnel: [w317 w322] -> w311
      tunnel: w308 -> [_ w324]
      tunnel: w307 -> [_ w323]
      frame False {
        n155 = Tick Count (ms)() -> (millisecond timer value=w321:u32)
        n156 = call "Read Drive Operation.vi"() -> ("Command Info"=w315:T25, "SubSystem Data"=w314:T3)  [unwired: 9 in, 1 out]
        n157 = Unbundle(w314) -> ("Operation"=w319:T4, "Left Speed"=w316:dbl)  [unwired: 9 out]
        n158 = Unbundle(w315) -> ("Status"=w318:T6)  [unwired: 2 out]
        n159 = Subtract(x=w321, y=w319) -> (x-y=w320:u32)
        n160 = Bundle(w320, "Left Speed"=w316) -> (w317:cluster{u32, "Left Speed":dbl})  [unwired: 1 in]
      }
      frame True {
        n161 = call "Drive Command Helper.vi"("Description"=w324, "SubSystem Data"=w323) -> ("Command Info Out"=w325:T25, "Command Timing"=w322:cluster{"Start Time (ms)":u32, "Iterations":i32})  [unwired: 7 in, 1 out]
        n162 = Unbundle(w325) -> ("Status"=w326:T6)  [unwired: 2 out]
      }
    }
    "Status" <- w310
    "Command Timing" <- w311
    n163 = Wait (ms)(milliseconds to wait=u32 20) -> ()  [unwired: 1 out]
  }
